vi "Generate Session ID.vi"() -> (2 "Session ID":i32)   [LabVIEW 2013, in "MQTT Server.lvlib" / "Session.lvclass"]
uses:
  Session.lvclass
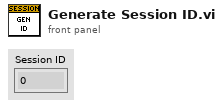
[diagram p1: front panel]
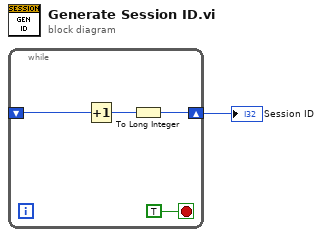
[diagram p0: block diagram]
diagram:
  n1 = while {
    shift-right: [w2] -> w1
    shift-left: _ -> [w4]
    stop <- TRUE stop-if-true
    n2 = Increment(x=w4) -> (x+1=w3:i32)
    n3 = To Long Integer(number=w3) -> (32bit integer=w2:i32)
  }
  "Session ID" <- w1
